vi "Shoot(Aimbot).vi"(4 "VisionPrepButton":bool, 6 "LowerButton":bool, 7 "Override Data":T1={"SpinupDuration(10ms)"=100, "ShotDuration(10ms)"=100, "PowerScale"=1.0, "AngleShift"=0}, 8 "error in":errorcluster, 9 "Collection Trigger":bool, 10 "Vision Distance":dbl, 11 "Trigger":bool) -> (0 "error out":errorcluster, 2 "LaunchSpeed(t/100ms)":dbl, 3 "AngleMotorPosition(t)":dbl)   [LabVIEW 2015]
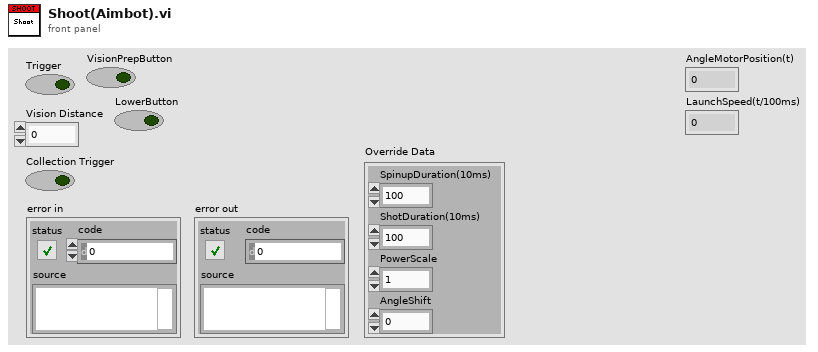
[diagram p1: front panel]
types:
  T1 = cluster{"SpinupDuration(10ms)":i32, "ShotDuration(10ms)":i32, "PowerScale":dbl, "AngleShift":i32}
  T2 = typedef "Bundle.ctl" = cluster{"error":errorcluster, "AngleMotorRefnum":T3, "LeftWheelRefnum":T3, "RightWheelRefnum":T3, "PushSolenoidRefnum":T10, "AngleMotorPosition(t)":dbl, "LaunchSpeed(t/100ms)":dbl, "CollectSpeed(t/100ms)":dbl, "SpinupDuration(10ms)":i32, "ShotDuration(10ms)":i32, "PowerScale":dbl, "AngleShift":i32, "VisionPrepAngle":dbl}
  T3 = typedef "WPI_MotorControlDeviceRef.ctl" = cluster{"DeviceStatus":errorcluster, "Type":T4, "PWM":cluster{"PWM Channel":T5, "DeadBand":T6}, "CAN":cluster{"Device Number":u8, "Control Mode":T7, "Semaphore":T8, "Max Vout":dbl, "TalonSRX Control Mode":T9}, "Invert":bool}
  T4 = typedef "WPI_MotorControlType.ctl" = enum16{"PWM", "CAN", "CANTalonSRX"}
  T5 = typedef "FPGA_DIOPWMChannel.ctl" = enum8{"PWM 0", "PWM 1", "PWM 2", "PWM 3", "PWM 4", "PWM 5", "PWM 6", "PWM 7", "PWM 8", "PWM 9", "PWM MXP 0", "PWM MXP 1", "PWM MXP 2", "PWM MXP 3", "PWM MXP 4", "PWM MXP 5", "PWM MXP 6", "PWM MXP 7", "PWM MXP 8", "PWM MXP 9", "Invalid"}
  T6 = typedef "WPI_PWMDeadband.ctl" = cluster{"Name":string, "maxPositivePwm":i32, "minPositivePwm":i32, "centerPwm":i32, "maxNegativePwm":i32, "minNegativePwm":i32, "angularRange":u16}
  T7 = typedef "WPI_CANJaguar_ControlMode.ctl" = enum8{"Percent VBus", "Current", "Speed", "Position", "Voltage"}
  T8 = typedef "Semaphore RefNum" = refnum<k1>
  T9 = typedef "WPI_CANTalonSRX_APIControlMode.ctl" = enum8{"Percent VBus", "Speed", "Position", "Slave", "Unchanged / Invalid", "Voltage Compensation", "Current", "Motion Profile"}
  T10 = typedef "WPI_SolenoidDevRef.ctl" = cluster{"DevStatus":errorcluster, "Pneumatics Control Module":u8, "Forward Solenoid Channel":T11, "Reverse Solenoid Channel":T11}
  T11 = typedef "WPI_SolenoidChannel.ctl" = enum8{"Solenoid 0", "Solenoid 1", "Solenoid 2", "Solenoid 3", "Solenoid 4", "Solenoid 5", "Solenoid 6", "Solenoid 7", "Invalid"}
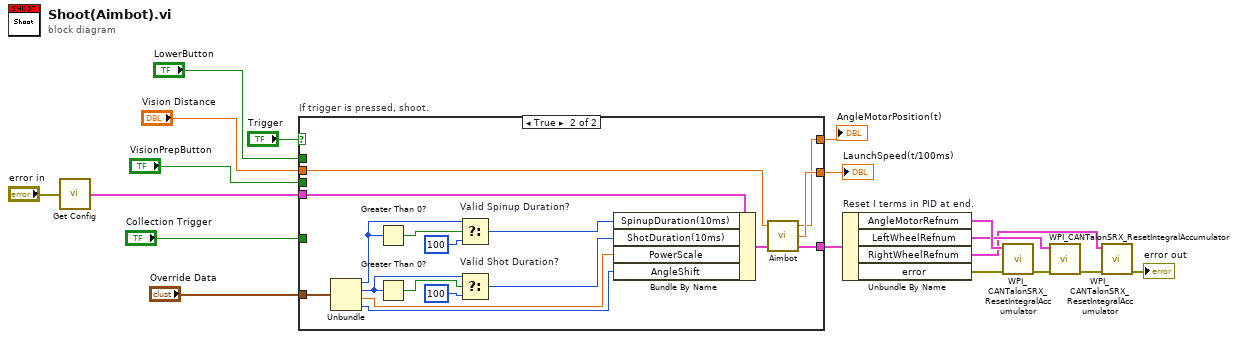
[diagram p0: block diagram]
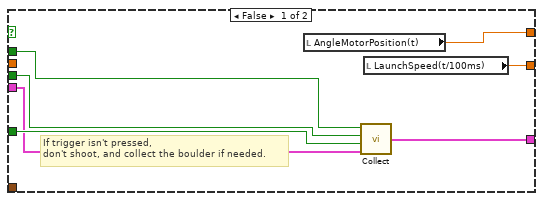
[diagram p2: hidden frame]
diagram:
  n1 = call "Get Config.vi"("error in"="error in") -> (0:w12:T2)
  n2 = case "If trigger is pressed, shoot." shown="True" "Trigger" {
    tunnel: [w23 w42] -> w8
    tunnel: "Vision Distance" -> [_ w41]
    tunnel: "Collection Trigger" -> [w25 _]
    tunnel: w12 -> [w24 w40]
    tunnel: "LowerButton" -> [w22 _]
    tunnel: "VisionPrepButton" -> [w21 _]
    tunnel: "Override Data" -> [_ w32]
    tunnel: [w20 w27] -> w2
    tunnel: [w19 w26] -> w1
    frame False {
      # "If trigger isn't pressed,\ndon't shoot, and collect the boulder if needed."
      n3 = local read "AngleMotorPosition(t)"() -> (w19:dbl)
      n4 = call "Collect.vi"("Firing Data"=w24, "CollectionTrigger"=w25, "VisionPrepButton"=w21, "LowerButton"=w22) -> ("Firing Data"=w23:T2)
      n5 = local read "LaunchSpeed(t/100ms)"() -> (w20:dbl)
    }
    frame True {
      n6 = Unbundle(w32) -> ("SpinupDuration(10ms)"=w31:i32, "ShotDuration(10ms)"=w30:i32, "PowerScale"=w29:dbl, "AngleShift"=w28:i32)
      n7 = Greater Than 0?(x=w31) -> (x > 0?=w35:bool)
      n8 = Greater Than 0?(x=w30) -> (x > 0?=w38:bool)
      n9 = Select "Valid Spinup Duration?"(t=w31, s=w35, f=100) -> (s? t:f=w33:i32)
      n10 = Select "Valid Shot Duration?"(t=w30, s=w38, f=100) -> (s? t:f=w36:i32)
      n11 = Bundle By Name(cluster=w40, "SpinupDuration(10ms)"=w33, "ShotDuration(10ms)"=w36, "PowerScale"=w29, "AngleShift"=w28) -> (w39:T2)
      n12 = call "Aimbot.vi"("Firing Data"=w39, "Range"=w41) -> ("Firing Data out"=w42:T2, "LaunchSpeed(t/100ms)"=w27:dbl, "AngleMotorPosition(t)"=w26:dbl)  [unwired: 1 in]
    }
  }
  "AngleMotorPosition(t)" <- w1
  "LaunchSpeed(t/100ms)" <- w2
  n13 = Unbundle By Name "Reset I terms in PID at end."(w8) -> ("AngleMotorRefnum"=w15:T3, "LeftWheelRefnum"=w14:T3, "RightWheelRefnum"=w13:T3, "error"=w7:errorcluster)
  n14 = call <vilib>:"WPI_CANTalonSRX_ResetIntegralAccumulator.vi"("error in (no error)"=w7, "CAN Talon SRX Ref"=w15) -> ("error out"=w17:errorcluster)  [unwired: 8 in, 1 out]
  n15 = call <vilib>:"WPI_CANTalonSRX_ResetIntegralAccumulator.vi"("error in (no error)"=w17, "CAN Talon SRX Ref"=w14) -> ("error out"=w18:errorcluster)  [unwired: 8 in, 1 out]
  n16 = call <vilib>:"WPI_CANTalonSRX_ResetIntegralAccumulator.vi"("error in (no error)"=w18, "CAN Talon SRX Ref"=w13) -> ("error out"=→"error out":errorcluster)  [unwired: 8 in, 1 out]
